vi "Configure.vi"(8 "error in (no error)":errorcluster, 10 "Network Stream Writer IP":string, 11 "DataReceiver in":refnum<class "DataReceiver.lvclass">) -> (0 "error out":errorcluster, 3 "DataReceiver out":refnum<class "DataReceiver.lvclass">)   [LabVIEW 2010, in "DataReceiver.lvclass"]
uses:
  DataReceiver.lvclass
  DataReceiver.lvclass/DataReceiver.ctl
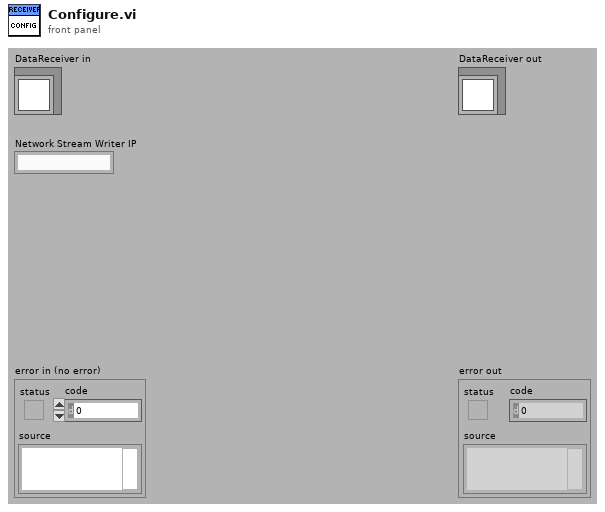
[diagram p1: front panel]
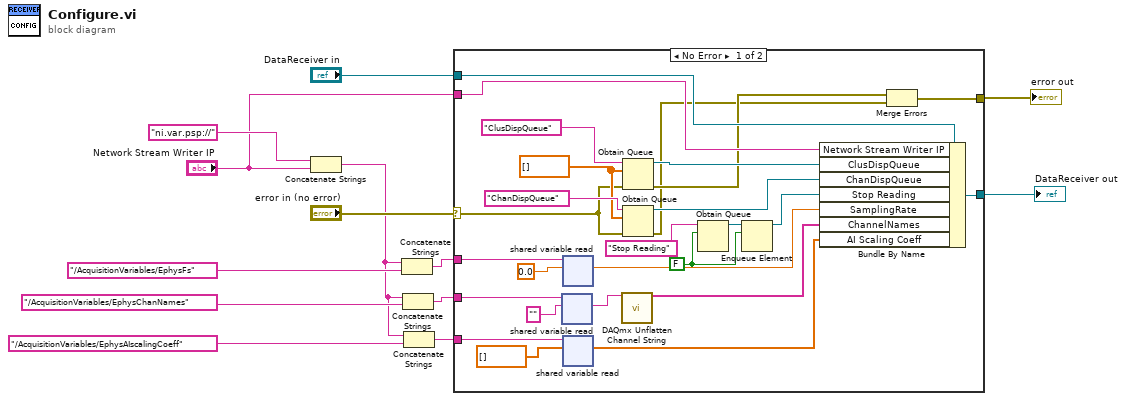
[diagram p0: block diagram]
diagram:
  n1 = Concatenate Strings("ni.var.psp://" ("string"), "Network Stream Writer IP") -> (w1:string)
  n2 = Concatenate Strings(w1, "/AcquisitionVariables/EphysFs" ("string")) -> (w7:string)
  n3 = Concatenate Strings(w1, "/AcquisitionVariables/EphysChanNames" ("string")) -> (w9:string)
  n4 = Concatenate Strings(w1, "/AcquisitionVariables/EphysAIscalingCoeff" ("string")) -> (w2:string)
  n5 = case shown="No Error" "error in (no error)" {
    selector: "error in (no error)" -> [w25 w41]
    tunnel: [w29 w41] -> w12
    tunnel: [w33 w40] -> w10
    tunnel: "DataReceiver in" -> [w38 w40]
    tunnel: "Network Stream Writer IP" -> [w32 _]
    tunnel: w9 -> [w23 _]
    tunnel: w7 -> [w24 _]
    tunnel: w2 -> [w22 _]
    frame No Error {
      w15 = FALSE ("element")
      w28 = dbl[] []
      n6 = shared-variable-read(w23, "") -> (w18:string)  [unwired: 1 in, 3 out]
      n7 = shared-variable-read(w24, 0.0) -> (w27:dbl)  [unwired: 1 in, 3 out]
      n8 = shared-variable-read(w22, dbl[] []) -> (w20:dbl[])  [unwired: 1 in, 3 out]
      n9 = call <vilib>:"DAQmx Unflatten Channel String.vi"("names in"=w18) -> ("names out"=w26:string[])  [unwired: 13 in, 1 out]
      n10 = Obtain Queue(name (unnamed)="ClusDispQueue", element data type=w28, error in (no error)=w25) -> (queue out=w35:refnum<queue>, error out=w31:errorcluster)  [unwired: 2 in, 1 out]
      n11 = Obtain Queue(name (unnamed)="ChanDispQueue", element data type=w28, error in (no error)=w25) -> (queue out=w34:refnum<queue>, error out=w30:errorcluster)  [unwired: 2 in, 1 out]
      n12 = Obtain Queue(name (unnamed)="Stop Reading", element data type=w15) -> (queue out=w17:refnum<queue>)  [unwired: 3 in, 2 out]
      n13 = Enqueue Element(queue=w17, element=w15) -> (queue out=w16:refnum<queue>)  [unwired: 2 in, 2 out]
      n14 = Bundle By Name(cluster=w38, "Network Stream Writer IP"=w32, "ClusDispQueue"=w35, "ChanDispQueue"=w34, "Stop Reading"=w16, "SamplingRate"=w27, "ChannelNames"=w26, "AI Scaling Coeff"=w20) -> (w33:refnum<class "DataReceiver.lvclass">)
      n15 = Merge Errors(w31, w30) -> (w29:errorcluster)
    }
    frame Error {
    }
  }
  "error out" <- w12
  "DataReceiver out" <- w10
